vi "TESTPanelHelper.vi"() -> ()   [LabVIEW 2009]
panel:
  in  "Cluster":errorcluster={"status"=TRUE, "code"=42, "source"="Error 42"}
  in  "Array":dbl[](array[numeric])=[0.0, 2.0, 3.0]
  in  "String":string="STRING"
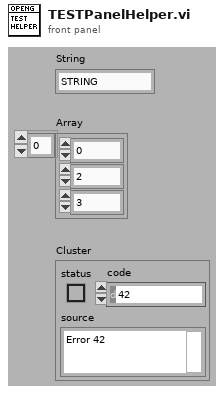
[diagram p1: front panel]
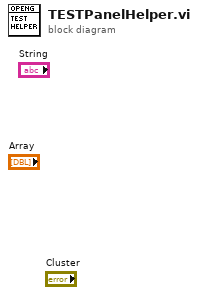
[diagram p0: block diagram]
diagram:
